vi "my_Color Wiener Filter.vi"() -> ()   [LabVIEW 2012]
doc: "This example showing the use case of Wiener Filter in imageprocessing. Wiener filter is a method of restoring image in the presence of blur (and noise) in the case when the blur kernel is known. In the given example I using Gaussian blur. This algorithm also can be used from restoring “motion blurred” images.\n\nA blurred or degraded image can be approximately described by equation Dst(x,y) = PSF * Src(x,y), where Src and Dst are source and result images and PSF is distortion operator called Point Spread Function. The Wiener filter can be understood better in the frequency domain. For deconvolution we will perform Fourier Transform of the blurred image, then perform convolution with inversed PSF function, and after inverse Fourier transform we will get the original image. When you know the exact PSF, the results of deblurring can be really effective."
uses:
  <vilib>/Analysis/2dsp.llb/2D Real FFT.vi
  <vilib>/Analysis/2dsp.llb/2D Inverse Real FFT.vi
  <vilib>/Analysis/NI_AALPro.lvlib
panel:
  out "image from file":picture
  out "initialized array 2":u32[][](array[numeric])
  out "blurred Image Size":i32[](array[numeric])
  out "path":path
  in  "path to JPEG file":path
  in  "Blurred Image - Lenna":dbl[][][](array[numeric])=array3x256x256[196608 elements]
  in  "Sigma":dbl=3.0 min=1.0 max=3.0 step=0.1 format="%_3g"
  out "Dst image (reconstructed)":picture
  out "Source image (blurred)":picture
  # "Wiener"
  # "Filter"
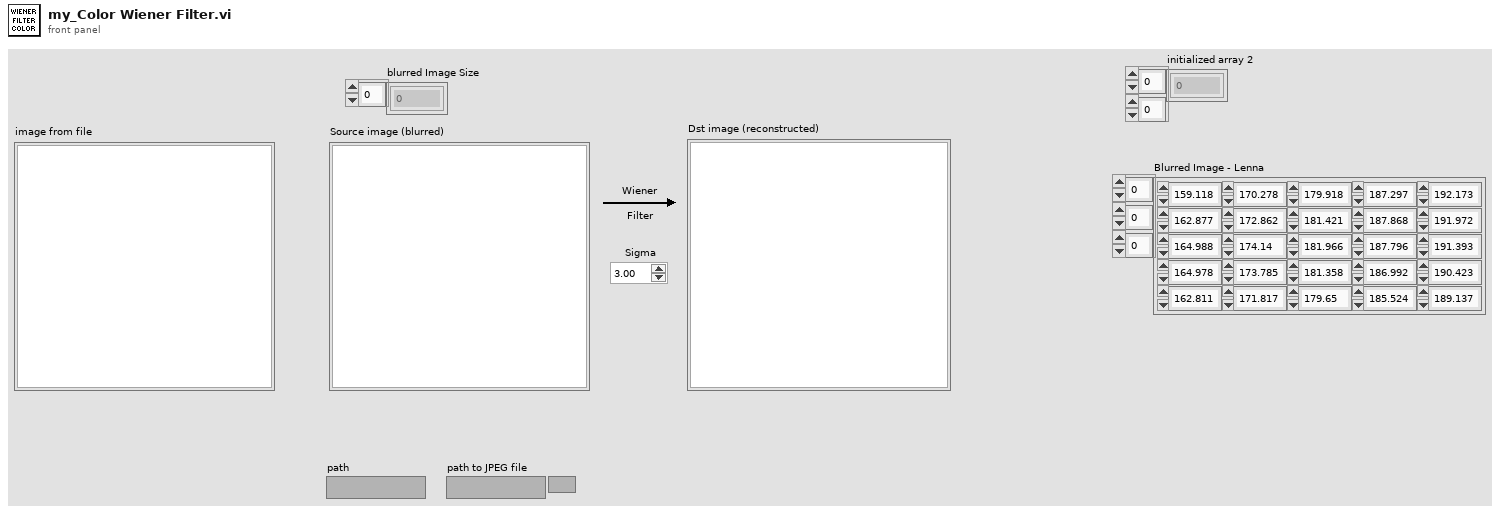
[diagram p1: front panel]
types:
  T1 = typedef "imagedata.ctl" = cluster{"image type":i32, "image depth":i32, "image":u8[], "mask":u8[], "colors":u32[], "Rectangle":cluster{"left":i16, "top":i16, "right":i16, "bottom":i16}}
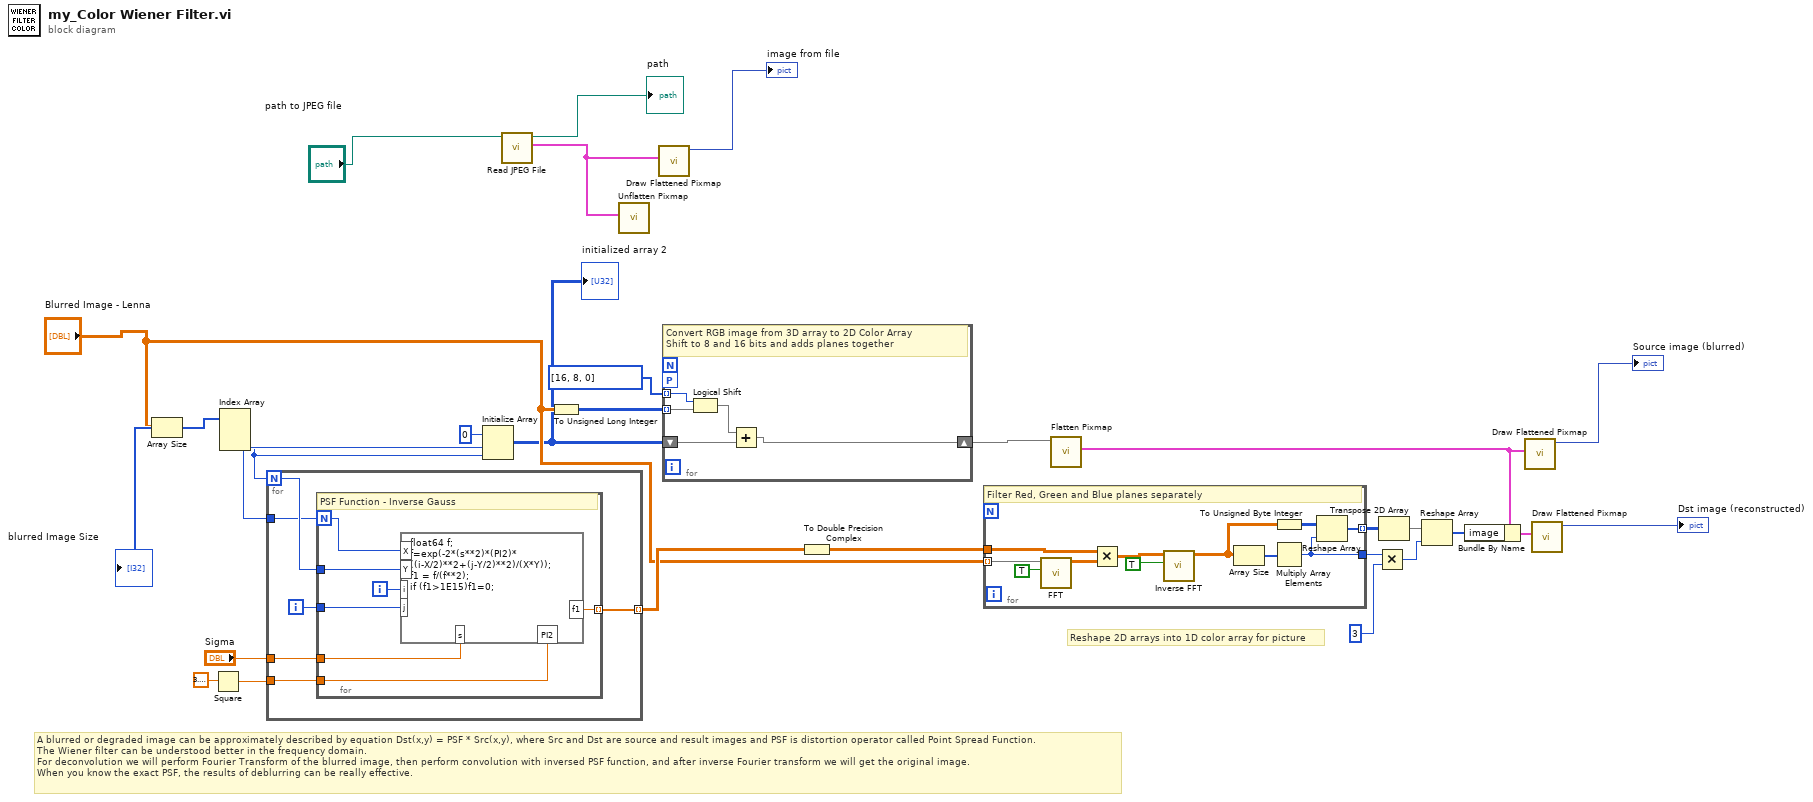
[diagram p0: block diagram]
diagram:
  # "A blurred or degraded image can be approximately described by equation Dst(x,y) = PSF * Src(x,y), where Src and Dst are source and result images and PSF is distortion operator called Point Spread Function.\nThe Wiener filter can be understood better in the frequency domain.\nFor deconvolution we will perform Fourier Transform of the blurred image, then perform convolution with inversed PSF function, and after inverse Fourier transform we will get the original image.\nWhen you know the exact PSF, the results of deblurring can be really effective."
  # "Reshape 2D arrays into 1D color array for picture"
  n1 = Array Size(array="Blurred Image - Lenna") -> (size(s)=w16:i32[])
  "blurred Image Size" <- w16
  n2 = Square(x=3.141592653589793) -> (x^2=w7:dbl)
  n3 = Index Array(array=w16) -> (element #2=w14:i32, element #3=w13:i32)  [unwired: 3 in, 1 out]
  n4 = for {
    N: w13 -> [w33]
    tunnel: "Sigma" -> [w34]
    tunnel: [w31] -> w10 mode=indexing
    tunnel: w14 -> [w30]
    tunnel: w7 -> [w29]
    i -> [w32]
    n5 = for {
      N: w30 -> [w40]
      tunnel: w34 -> [w41]
      tunnel: w33 -> [w39]
      tunnel: w32 -> [w37]
      tunnel: [w36] -> w31 mode=indexing
      tunnel: w29 -> [w35]
      i -> [w38]
      # "PSF Function - Inverse Gauss"
      n6 = formula code="float64 f;\nf=exp(-2*(s**2)*(PI2)*\n((i-X/2)**2+(j-Y/2)**2)/(X*Y));\nf1 = f/(f**2);\nif (f1>1E15)f1=0;"("s"=w41, "X"=w40, "i"=w38, "j"=w37, "PI2"=w35, "Y"=w39) -> ("f1"=w36:dbl)
    }
  }
  n7 = Initialize Array(u32 0 ("dimension size"), w14, w13) -> (w3:u32[][])
  "initialized array 2" <- w3
  n8 = call <vilib>:"Read JPEG File.vi"("path to JPEG file"="path to JPEG file") -> ("image data"=w1:T1, "path"=→"path":path)  [unwired: 8 in, 1 out]
  n9 = To Unsigned Long Integer(number="Blurred Image - Lenna") -> (unsigned 32bit integer=w21:u32[][][])
  n10 = call <vilib>:"Unflatten Pixmap.vi"("image data"=w1) -> ()  [unwired: 4 in, 7 out]
  n11 = call <vilib>:"Draw Flattened Pixmap.vi"("image data"=w1) -> ("new picture"=→"image from file":picture)  [unwired: 8 in]
  n12 = for {
    tunnel: w21 -> [w45] mode=indexing
    shift-right: [w46] -> w19
    shift-left: w3 -> [w44]
    tunnel: i32[] [16, 8, 0] ("unsharp image") -> [w42] mode=indexing
    workers-P: _ -> [_]
    # "Convert RGB image from 3D array to 2D Color Array\nShift to 8 and 16 bits and adds planes together"
    n13 = Logical Shift(y=w42, x=w45) -> (x << y=w43:u32[][])
    n14 = Add(x=w43, y=w44) -> (x+y=w46:u32[][])
  }
  n15 = To Double Precision Complex(1:w10) -> (0:w9:cdb[][])
  n16 = for {
    tunnel: [w53] -> w27 mode=indexing
    tunnel: [w52] -> w23
    tunnel: "Blurred Image - Lenna" -> [w51] mode=indexing
    tunnel: w9 -> [w49]
    # "Filter Red, Green and Blue planes separately"
    n17 = call-poly <vilib>:"FFT.vi"("shift?"=TRUE, "X"=w51) -> ("FFT {X}"=w47:cdb[][])  [unwired: 8 in, 1 out]
    n18 = Multiply(x=w49, y=w47) -> (x*y=w50:cdb[][])
    n19 = call-poly <vilib>:"Inverse FFT.vi"("shift?"=TRUE, "FFT {X}"=w50) -> ("X"=w54:dbl[][])  [unwired: 8 in, 1 out]
    n20 = Array Size(array=w54) -> (size(s)=w55:i32[])
    n21 = To Unsigned Byte Integer(number=w54) -> (unsigned 8bit integer=w48:u8[][])
    n22 = Multiply Array Elements(1:w55) -> (0:w52:i32)
    n23 = Reshape Array(w48, w52) -> (w53:u8[])
  }
  n24 = call <vilib>:"Flatten Pixmap.vi"("24-bit pixmap"=w19) -> ("image data"=w18:T1)  [unwired: 10 in]
  n25 = Multiply(x=w23, y=3 ("x")) -> (x*y=w26:i32)
  n26 = Transpose 2D Array(2D array=w27) -> (transposed array=w24:u8[][])
  n27 = Reshape Array(w24, w26) -> (w25:u8[])
  n28 = Bundle By Name(cluster=w18, "image"=w25) -> (w28:T1)
  n29 = call <vilib>:"Draw Flattened Pixmap.vi"("image data"=w18) -> ("new picture"=→"Source image (blurred)":picture)  [unwired: 8 in]
  n30 = call <vilib>:"Draw Flattened Pixmap.vi"("image data"=w28) -> ("new picture"=→"Dst image (reconstructed)":picture)  [unwired: 8 in]
